vi "Multiple Connections - Server.vi"() -> ()   [LabVIEW 2016]
doc: "Demonstrates how to establish multiple connections and place them in a queue to be serviced. As connections are made, it sends the current date and time via TCP to all Client VIs that connect to it.\n\nThis VI has two parts -- a loop that listens for each client to connect, and a loop that sends the date and time to each connection in the queue.\n\n<B>Note:</B> Use this VI with Multiple Connections - Client 1.vi and Multiple Connections - Client 2.vi."
panel:
  in  "listen halted":bool
  in  "stop":bool
  out "# of Connections":i32
  in  "empty":refnum<k5>[](array[refnum])
  in  "empty":refnum<k5>[](array[refnum])
  in  "Port":u16=6341
  # "Instructions:\n1. Open the Multiple Connections - Client 1 and Client 2 VIs.\n2. Run this VI first.\n3. Run the Client VIs second and follow the instructions on their front panels.\n4. Stop This VI.  The Client VIs will stop on their own when they time out."
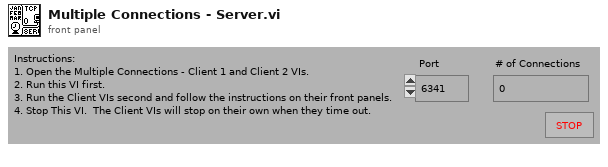
[diagram p1: front panel]
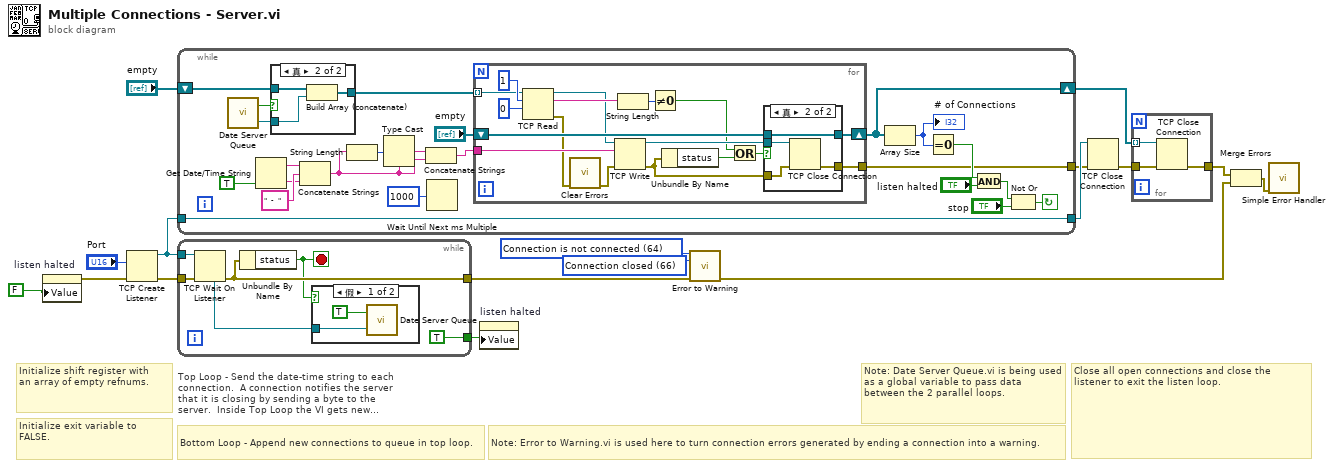
[diagram p0: block diagram]
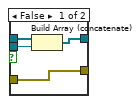
[diagram p2: hidden frame]
diagram:
  w9 = 66 items=["No Error", "Argument Error", "Memory Full", "Out of Zone", "End of File", "File Already Open", "Generic File IO Error", "File Not Found", "File Permission Error", "Disk Full", "Duplicate Path", "Too Many Files Open", "Not Enabled", "Resource File Not Found", "Cannot Add Resource", "Resource Not Found", "Image Not Found", "Image Memory Error", "Pen Does Not Exist", "Config Bad Type", "Config Token Not Found", "Config Parse Error", "Config Memory Error", "Bad External Code Format", "Bad External Code Offset", "External Code Not Present", "Null Window", "Destroy Window Mixup", "Null Menu", "Print Aborted", "Bad Print Record", "Print Driver Error", "Windows Error During Print", "Memory Error During Print", "Print Dialog Error", "Generic Print Error", "Invalid Device Refnum", "Device Not Found", "Device Parameter Error", "Device Unit Error", "Can't Open Device", "Device Call Aborted", "Generic Error", "Cancelled By User", "Object ID Too Low", "Object ID Too High", "Object Not In Heap", "Unknown Heap", "Bad DefProc ID", "DefProc Not In Table", "Message Out Of Range", "Null Method", "Unknown Message", "Manager Call Not Supported", "Bad address", "Connection In progress", "Connection timed out", "Connection is already in progress", "Network attribute not supported", "Network error", "Address in use", "System out of memory", "Connection aborted", "Connection refused", "Connection is not connected", "Connection is already connected", "Connection closed", "Initialize error (interapplication manager)", "Bad occurrence", "Wait on unbound occurrence handler", "Occurrence queue overflow", "Bad path", "Semaphore not signaled", "Unrecognized type (interapplication manager)"] ("2nd Error to Convert")
  w10 = 64 items=["No Error", "Argument Error", "Memory Full", "Out of Zone", "End of File", "File Already Open", "Generic File IO Error", "File Not Found", "File Permission Error", "Disk Full", "Duplicate Path", "Too Many Files Open", "Not Enabled", "Resource File Not Found", "Cannot Add Resource", "Resource Not Found", "Image Not Found", "Image Memory Error", "Pen Does Not Exist", "Config Bad Type", "Config Token Not Found", "Config Parse Error", "Config Memory Error", "Bad External Code Format", "Bad External Code Offset", "External Code Not Present", "Null Window", "Destroy Window Mixup", "Null Menu", "Print Aborted", "Bad Print Record", "Print Driver Error", "Windows Error During Print", "Memory Error During Print", "Print Dialog Error", "Generic Print Error", "Invalid Device Refnum", "Device Not Found", "Device Parameter Error", "Device Unit Error", "Can't Open Device", "Device Call Aborted", "Generic Error", "Cancelled By User", "Object ID Too Low", "Object ID Too High", "Object Not In Heap", "Unknown Heap", "Bad DefProc ID", "DefProc Not In Table", "Message Out Of Range", "Null Method", "Unknown Message", "Manager Call Not Supported", "Bad address", "Connection In progress", "Connection timed out", "Connection is already in progress", "Network attribute not supported", "Network error", "Address in use", "System out of memory", "Connection aborted", "Connection refused", "Connection is not connected", "Connection is already connected", "Connection closed", "Initialize error (interapplication manager)", "Bad occurrence", "Wait on unbound occurrence handler", "Occurrence queue overflow", "Bad path", "Semaphore not signaled", "Unrecognized type (interapplication manager)"] ("1st Error to Convert")
  # "Note: Date Server Queue.vi is being used as a global variable to pass data between the 2 parallel loops."
  # "Note: Error to Warning.vi is used here to turn connection errors generated by ending a connection into a warning."
  # "Initialize shift register with\nan array of empty refnums."
  # "Bottom Loop - Append new connections to queue in top loop."
  # "Initialize exit variable to FALSE."
  # "Close all open connections and close the listener to exit the listen loop."
  n1 = property on="listen halted" class="Bool (严格)"("Value"=FALSE) -> (error out=w5:errorcluster)  [unwired: 2 in, 1 out]
  n2 = TCP Create Listener(8:w5, 10:"Port") -> (0:w15:errorcluster, 3:w13:refnum<k5>)  [unwired: 4 out]
  n3 = while "Top Loop - Send the date-time string to each connection.  A connection notifies the server that it is closing by sending a byte to the server.  Inside Top Loop the VI gets new connections one at a time from the queue.  The listen halted control is a hidden control.  It is used to notify the work loop that the listener (bottom loop) has halted.  The top loop will stop if the listener is halted or the stop button is pressed." {
    shift-left: "empty" -> [w38]
    shift-right: [w29] -> w17
    tunnel: w13 -> [w19]
    tunnel: [w19] -> w14
    tunnel: [w18] -> w4
    stop <- w21 continue-if-true
    n4 = call "Date Server Queue.vi"() -> ("value"=w40:refnum<k5>, "valid?"=w39:bool)  [unwired: 2 in]
    n5 = Get Date/Time String(want seconds? (F)=TRUE) -> (date string=w34:string, time string=w26:string)  [unwired: 2 out]
    n6 = case shown="真" w39 {
      tunnel: w40 -> [_ w69]
      tunnel: w38 -> [w66 w68]
      tunnel: [w66 w67] -> w36
      frame False {
      }
      frame True {
        n7 = Build Array (concatenate)(w68, w69) -> (w67:refnum<k5>[])
      }
    }
    n8 = Concatenate Strings(w34, "  -  ", w26) -> (w32:string)
    n9 = String Length(string=w32) -> (length=w33:i32)
    n10 = Type Cast(type=w32, x=w33) -> (*(type *) &x=w31:string)
    n11 = Concatenate Strings(w31, w32) -> (w30:string)
    n12 = Wait Until Next ms Multiple(millisecond multiple=u32 1000) -> ()  [unwired: 1 out]
    n13 = for {
      tunnel: w36 -> [w47] mode=indexing
      shift-right: [w54] -> w29
      shift-left: "empty" -> [w56]
      tunnel: w30 -> [w57]
      tunnel: [w41] -> w18
      n14 = TCP Read(connection ID=w47, bytes to read=1, 9:0) -> (connection ID out=w46:refnum<k5>, data out=w51:string, error out=w43:errorcluster)  [unwired: 1 in, 1 out]
      n15 = call <vilib>:"Clear Errors.vi"("error in (no error)"=w43) -> ("error out"=w42:errorcluster)  [unwired: 1 in, 5 out]
      n16 = TCP Write(connection ID=w46, data in=w57, error in (no error)=w42) -> (connection ID out=w55:refnum<k5>, error out=w44:errorcluster)  [unwired: 2 out]
      n17 = String Length(string=w51) -> (length=w50:i32)
      n18 = Not Equal To 0?(x=w50) -> (x != 0?=w48:bool)
      n19 = Unbundle By Name(w44) -> ("status"=w45:bool)
      n20 = Or(x=w48, y=w45) -> (x .or. y?=w49:bool)
      n21 = case shown="真" w49 {
        tunnel: w56 -> [w61 w65]
        tunnel: w55 -> [w60 w64]
        tunnel: [w59 w65] -> w54
        tunnel: w44 -> [w58 w63]
        tunnel: [w58 w62] -> w41
        frame False {
          n22 = Build Array (concatenate)(w61, w60) -> (w59:refnum<k5>[])
        }
        frame True {
          n23 = TCP Close Connection(connection ID=w64, error in (no error)=w63) -> (error out=w62:errorcluster)  [unwired: 2 out]
        }
      }
    }
    n24 = Array Size(array=w29) -> (size(s)=w24:i32)
    "# of Connections" <- w24
    n25 = Equal To 0?(x=w24) -> (x = 0?=w25:bool)
    n26 = And(x=w25, y="listen halted") -> (x .and. y?=w22:bool)
    n27 = Not Or(1:"stop", 2:w22) -> (0:w21:bool)
  }
  n28 = while "Listen loop.  Append new connections to a synchronized queue." {
    tunnel: w13 -> [w74]
    tunnel: w15 -> [w75]
    tunnel: [w72] -> w11
    tunnel: [TRUE] -> w12
    stop <- w71 stop-if-true
    n29 = TCP Wait On Listener(8:w75, 11:w74) -> (0:w72:errorcluster, 4:w73:refnum<k5>)  [unwired: 5 out]
    n30 = Unbundle By Name(w72) -> ("status"=w71:bool)
    n31 = case shown="假" w71 {
      tunnel: w73 -> [w76 _]
      frame False {
        n32 = call "Date Server Queue.vi"("new value"=w76, "set queue? (F: de-queue)"=TRUE) -> ()  [unwired: 2 out]
      }
      frame True {
      }
    }
  }
  n33 = property on="listen halted" class="Bool (严格)"("Value"=w12) -> ()  [unwired: 2 in, 2 out]
  n34 = call <vilib>:"Error to Warning.vi"("1st Error to Convert"=w10, "2nd Error to Convert"=w9, "error in"=w11) -> ("warning out"=w2:errorcluster)  [unwired: 2 in, 10 out]
  n35 = TCP Close Connection(connection ID=w14, error in (no error)=w4) -> (error out=w3:errorcluster)  [unwired: 2 out]
  n36 = for {
    tunnel: w17 -> [w80] mode=indexing
    tunnel: [w79] -> w8
    tunnel: w3 -> [w78]
    n37 = TCP Close Connection(connection ID=w80, error in (no error)=w78) -> (error out=w79:errorcluster)  [unwired: 2 out]
  }
  n38 = Merge Errors(w8, w2) -> (w7:errorcluster)
  n39 = call <vilib>:"Simple Error Handler.vi"("error in (no error)"=w7) -> ()  [unwired: 1 in, 8 out]
